vi "Conveyor Controls.vi"(11 "CTR to CMNDS":T1) -> ()   [LabVIEW 2014]
uses:
  JoyStick/Commands.ctl
  Global Variables/Refnums.vi
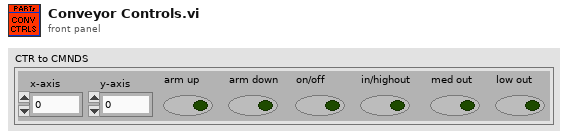
[diagram p1: front panel]
types:
  T1 = typedef "Commands.ctl" = cluster{"x-axis":dbl, "y-axis":dbl, "arm up":bool, "arm down":bool, "on/off":bool, "in/highout":bool, "med out":bool, "low out":bool}
  T2 = typedef "WPI_MotorControlDeviceRef.ctl" = cluster{"DeviceStatus":errorcluster, "Type":enum16{"PWM", "CAN"}, "PWM":cluster{"Digital Module":T3, "PWM Channel":T4, "DeadBand":T5}, "CAN":cluster{"Device Number":u8, "Control Mode":T6, "Semaphore":T7, "Max Vout":dbl}, "Invert":bool, "TransformRef":T8, "InvTransformRef":T8}
  T3 = typedef "FPGA_TypedefDigitalModule.ctl" = enum16{"Digital Module 1", "Digital Module 2"}
  T4 = typedef "FPGA_DIOPWMChannel.ctl" = enum8{"PWM 1", "PWM 2", "PWM 3", "PWM 4", "PWM 5", "PWM 6", "PWM 7", "PWM 8", "PWM 9", "PWM 10", "Invalid"}
  T5 = typedef "WPI_PWMDeadband.ctl" = cluster{"Name":string, "maxPositivePwm":i32, "minPositivePwm":i32, "centerPwm":i32, "maxNegativePwm":i32, "minNegativePwm":i32, "angularRange":u16}
  T6 = typedef "WPI_CANJaguar_ControlMode.ctl" = enum8{"Percent VBus", "Current", "Speed", "Position", "Voltage"}
  T7 = typedef "Semaphore RefNum" = refnum<k1>
  T8 = typedef "WPI_PWMTransform_ConPane.ctl" = refnum<vi>
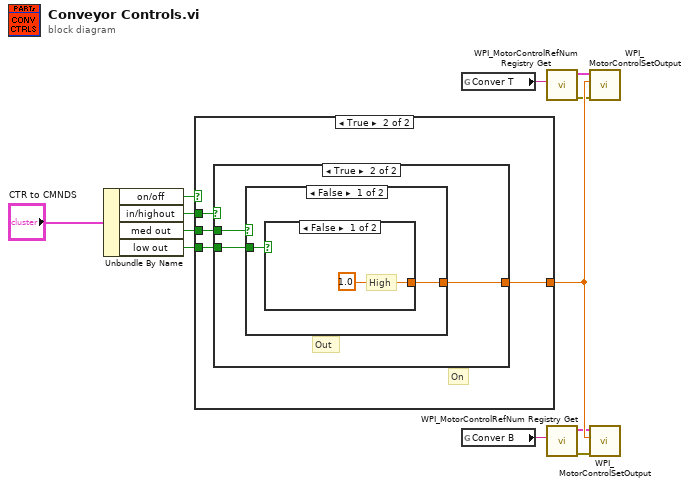
[diagram p0: block diagram]
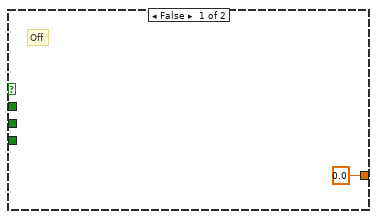
[diagram p2: hidden frame]
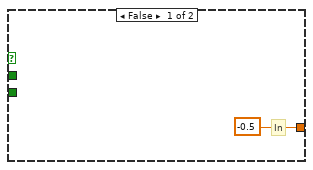
[diagram p3: hidden frame]
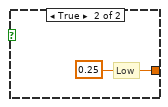
[diagram p4: hidden frame]
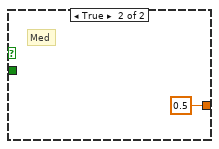
[diagram p5: hidden frame]
diagram:
  n1 = Unbundle By Name("CTR to CMNDS") -> ("on/off"=w8:bool, "in/highout"=w9:bool, "med out"=w10:bool, "low out"=w11:bool)
  n2 = case shown="True" w8 {
    tunnel: w9 -> [_ w17]
    tunnel: w10 -> [_ w16]
    tunnel: w11 -> [_ w15]
    tunnel: [0.0 w14] -> w12
    frame False {
      # "Off"
    }
    frame True {
      # "On"
      n3 = case shown="True" w17 {
        tunnel: w16 -> [_ w21]
        tunnel: w15 -> [_ w20]
        tunnel: [-0.5 w19] -> w14
        frame False {
          # "In"
        }
        frame True {
          # "Out"
          n4 = case shown="False" w21 {
            tunnel: w20 -> [w23 _]
            tunnel: [w22 0.5] -> w19
            frame False {
              n5 = case shown="False" w23 {
                tunnel: [1.0 0.25] -> w22
                frame False {
                  # "High"
                }
                frame True {
                  # "Low"
                }
              }
            }
            frame True {
              # "Med"
            }
          }
        }
      }
    }
  }
  n6 = global read "Refnums.vi" "Conver T"() -> (w5:string)
  n7 = global read "Refnums.vi" "Conver B"() -> (w6:string)
  n8 = call <vilib>:"WPI_MotorControlRefNum Registry Get.vi"("refnum name"=w5) -> ("error out"=w2:errorcluster, "MotorControlDevRef"=w1:T2)  [unwired: 9 in]
  n9 = call <vilib>:"WPI_MotorControlRefNum Registry Get.vi"("refnum name"=w6) -> ("error out"=w4:errorcluster, "MotorControlDevRef"=w3:T2)  [unwired: 9 in]
  n10 = call <vilib>:"WPI_MotorControlSetOutput.vi"("error in (no error)"=w2, "Output"=w12, "MotorControlDevRef"=w1) -> ()  [unwired: 6 in, 3 out]
  n11 = call <vilib>:"WPI_MotorControlSetOutput.vi"("error in (no error)"=w4, "Output"=w12, "MotorControlDevRef"=w3) -> ()  [unwired: 6 in, 3 out]
